vi "config channel.vi"(8 "error in":errorcluster, 11 "DAQ Config":T1) -> (0 "error out":errorcluster, 3 "DAQ Config out":T1)   [LabVIEW 2017]
uses:
  Control/Config chanel.ctl
  <vilib>/DAQmx/create/channels.llb/DAQmx Create Channel (AI-Voltage-Basic).vi
  <vilib>/DAQmx/configure/timing.llb/DAQmx Timing (Sample Clock).vi
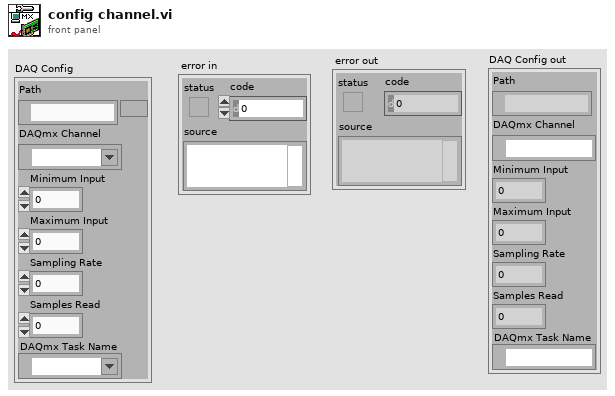
[diagram p1: front panel]
types:
  T1 = typedef "Config chanel.ctl" = cluster{"Path":path, "DAQmx Channel":tag, "Minimum Input":dbl, "Maximum Input":dbl, "Sampling Rate":dbl, "Samples Read":dbl, "DAQmx Task Name":refnum<k21>}
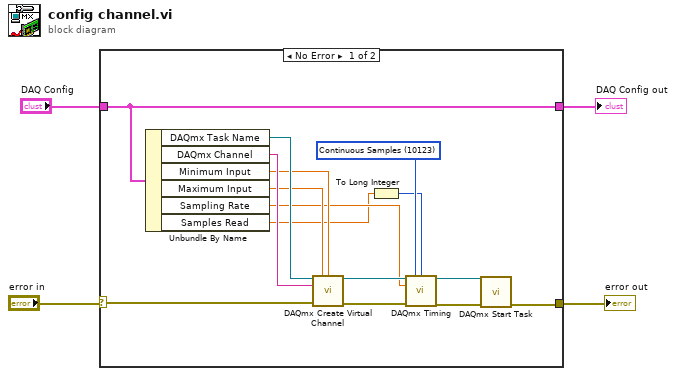
[diagram p0: block diagram]
diagram:
  n1 = case shown="No Error" "error in" {
    selector: "error in" -> [w5 w20]
    tunnel: [w10 w20] -> w4
    tunnel: [w19 w21] -> w2
    tunnel: "DAQ Config" -> [w19 w21]
    frame No Error {
      w9 = 10123 items=["Finite Samples"=10178, "Continuous Samples"=10123, "Hardware Timed Single Point"=12522] ("sample mode")
      n2 = Unbundle By Name(w19) -> ("DAQmx Task Name"=w18:refnum<k21>, "DAQmx Channel"=w17:tag, "Minimum Input"=w16:dbl, "Maximum Input"=w15:dbl, "Sampling Rate"=w8:dbl, "Samples Read"=w7:dbl)
      n3 = call-poly <vilib>:"DAQmx Create Virtual Channel.vi"("task in"=w18, "maximum value"=w15, "minimum value"=w16, "physical channels"=w17, "error in"=w5) -> ("task out"=w14:refnum<k21>, "error out"=w13:errorcluster)  [unwired: 9 in]
      n4 = To Long Integer(number=w7) -> (32bit integer=w6:i32)
      n5 = call-poly <vilib>:"DAQmx Timing.vi"("task/channels in"=w14, "sample mode"=w9, "samples per channel"=w6, "rate"=w8, "error in"=w13) -> ("task out"=w12:refnum<k21>, "error out"=w11:errorcluster)  [unwired: 9 in]
      n6 = call <vilib>:"DAQmx Start Task.vi"("task/channels in"=w12, "error in"=w11) -> ("error out"=w10:errorcluster)  [unwired: 12 in, 1 out]
    }
    frame Error {
    }
  }
  "DAQ Config out" <- w2
  "error out" <- w4
